vi "Get Class Data.vi"(7 "OwningVI":refnum<vi>, 11 "Class":variant) -> (2 "Can Access Members?":bool, 3 "Class Data":variant[](array[variant]))   [LabVIEW 2020, in "Better Search.lvlib"]
uses:
  Better Search.lvlib
  <vilib>/Utility/Data Type/NI_Data Type.lvlib
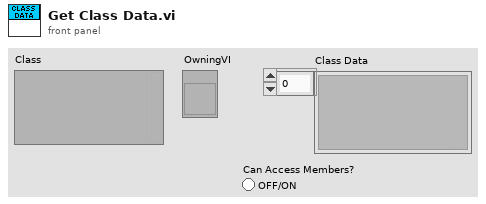
[diagram p1: front panel]
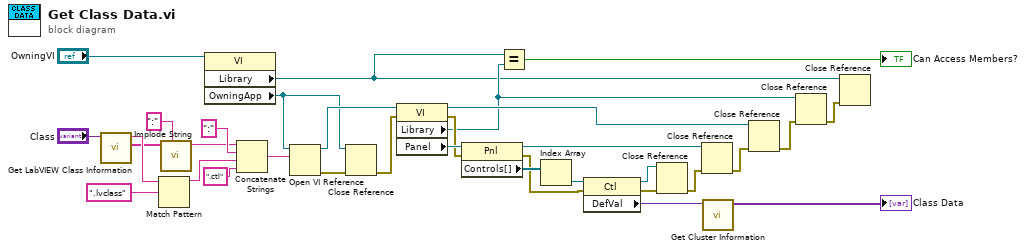
[diagram p0: block diagram]
diagram:
  n1 = call <vilib>:"Get LabVIEW Class Information.vi"("variant"="Class") -> ("qualified LabVIEW class name"=w3:string[], "LabVIEW class file name"=w6:string)  [unwired: 8 in, 1 out]
  n2 = Match Pattern(string=w6, regular expression=".lvclass") -> (before substring=w26:string)  [unwired: 1 in, 3 out]
  n3 = call "Implode String.vi"("Delimiter (Comma)"=":" ("delimiter"), "String Array"=w3) -> ("Delimited String"=w2:string)  [unwired: 9 in]
  n4 = property class="VI"(reference="OwningVI") -> ("Library"=w7:refnum<vi>, "OwningApp"=w21:refnum<vi>)  [unwired: 1 in, 2 out]
  n5 = Concatenate Strings(w2, ":" ("string"), w26, ".ctl" ("string")) -> (w20:string)
  n6 = Open VI Reference(application reference (local)=w21, vi path=w20) -> (vi reference=w24:refnum<vi>, error out=w23:errorcluster)  [unwired: 4 in]
  n7 = Close Reference(reference=w21, error in (no error)=w23) -> (error out=w22:errorcluster)
  n8 = property class="VI"(reference=w24, error in=w22) -> (reference out=w13:refnum<vi>, error out=w30:errorcluster, "Library"=w9:refnum<vi>, "Panel"=w33:refnum<vi>)
  n9 = property class="Pnl"(reference=w33, error in=w30) -> (reference out=w14:refnum<vi>, error out=w29:errorcluster, "Controls[]"=w32:refnum<vi>[])
  n10 = Equal?(x=w7, y=w9) -> (x = y?=→"Can Access Members?":bool)
  n11 = Index Array(array=w32) -> (element=w31:refnum<vi>)  [unwired: 1 in]
  n12 = property class="Ctl"(reference=w31, error in=w29) -> (reference out=w16:refnum<vi>, error out=w17:errorcluster, "DefVal"=w5:variant)
  n13 = Close Reference(reference=w16, error in (no error)=w17) -> (error out=w15:errorcluster)
  n14 = Close Reference(reference=w14, error in (no error)=w15) -> (error out=w12:errorcluster)
  n15 = call <vilib>:"Get Cluster Information.vi"("variant"=w5) -> ("cluster elements"=→"Class Data":variant[])  [unwired: 9 in, 1 out]
  n16 = Close Reference(reference=w13, error in (no error)=w12) -> (error out=w10:errorcluster)
  n17 = Close Reference(reference=w9, error in (no error)=w10) -> (error out=w8:errorcluster)
  n18 = Close Reference(reference=w7, error in (no error)=w8) -> ()  [unwired: 1 out]
